vi "Array Generation.vi"(1 "Number of Steps":dbl, 2 "Lower Bound":dbl, 3 "Upper Bound":dbl) -> (0 "Output Array":dbl[](array[numeric]))   [LabVIEW 2020]
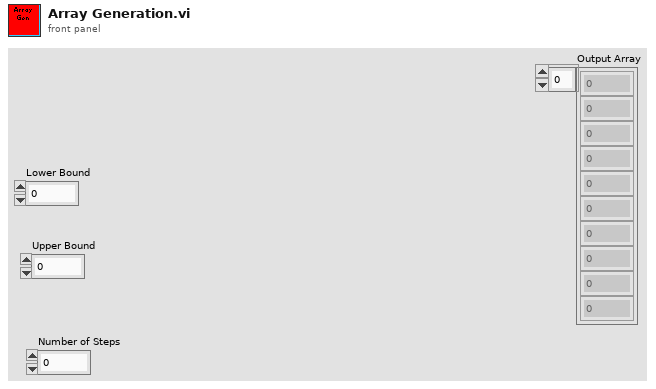
[diagram p1: front panel]
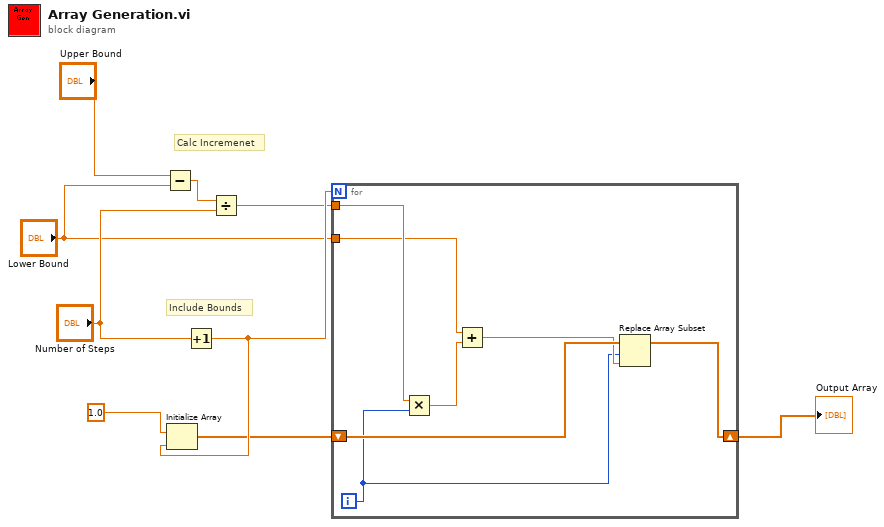
[diagram p0: block diagram]
diagram:
  # "Include Bounds"
  # "Calc Incremenet"
  n1 = Subtract(x="Upper Bound", y="Lower Bound") -> (x-y=w8:dbl)
  n2 = Increment(x="Number of Steps") -> (x+1=w5:dbl)
  n3 = Initialize Array(1.0, w5) -> (w4:dbl[])
  n4 = Divide(x=w8, y="Number of Steps") -> (x/y=w3:dbl)
  n5 = for {
    N: w5 -> [_]
    shift-right: [w10] -> w1
    shift-left: w4 -> [w13]
    tunnel: w3 -> [w16]
    tunnel: "Lower Bound" -> [w14]
    i -> [w11]
    n6 = Multiply(x=w16, y=w11) -> (x*y=w15:dbl)
    n7 = Add(x=w14, y=w15) -> (x+y=w12:dbl)
    n8 = Replace Array Subset(array=w13, new element=w12, index=w11) -> (w10:dbl[])
  }
  "Output Array" <- w1
